vi "Configure Meas Complete Dest [MP].vi"(8 "error in (no error)":errorcluster, 10 "meas complete dest (None)":i32(ring)=-1 items=["None"=-1, "External"=2, "PXI TRIG0 or VXI TTL0"=111, "PXI TRIG1 or VXI TTL1"=112, "PXI TRIG2 or VXI TTL2"=113, "PXI TRIG3 or VXI TTL3"=114, "PXI TRIG4 or VXI TTL4"=115, "PXI TRIG5 or VXI TTL5"=116, "PXI TRIG6 or VXI TTL6"=117, "PXI TRIG7 or VXI TTL7"=118, "ECL0"=119, "ECL1"=120, "PXI Star"=131, "RTSI 0"=140, "RTSI 1"=141, "RTSI 2"=142, "RTSI 3"=143, "RTSI 4"=144, "RTSI 5"=145, "RTSI 6"=146], 11 "CS++DMM in":refnum<class "CS++DMM.lvclass">) -> (0 "error out":errorcluster, 3 "CS++DMM out":refnum<class "CS++DMM.lvclass">)   [LabVIEW 2013, in "CS++DMM.lvlib" / "CS++DMM.lvclass"]
doc: "This VI configures the destination of the measurement-complete signal. This signal is commonly referred to as Voltmeter Complete.\n\nNote:\n\n(1) This VI is part of the IviDmmMultiPoint [MP] extension group."
uses:
  CS++DMM.lvclass
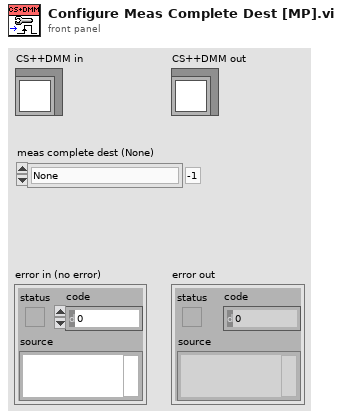
[diagram p1: front panel]
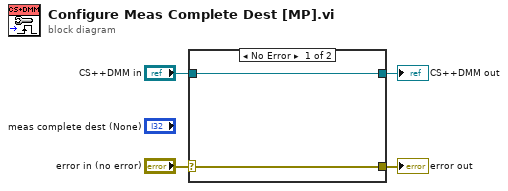
[diagram p0: block diagram]
diagram:
  n1 = case shown="No Error" "error in (no error)" {
    selector: "error in (no error)" -> [w5 w8]
    tunnel: [w5 w8] -> w3
    tunnel: [w6 w7] -> w1
    tunnel: "CS++DMM in" -> [w6 w7]
    frame No Error {
    }
    frame Error {
    }
  }
  "error out" <- w3
  "CS++DMM out" <- w1
